vi "PH_Beckhoff.scale analog Beckhoff Value.vi"(0 "Beckhoff value":u32, 1 "Scaling Type":T1) -> (2 "DIM value":dbl)   [LabVIEW 2014, in "PH_Beckhoff.lvlib"]
doc: "This VI is forseen to scale the raw digital Beckhoff value to the DIM value to be published."
uses:
  PH_Beckhoff.lvlib
  PH_Beckhoff.Scaling Type.ctl
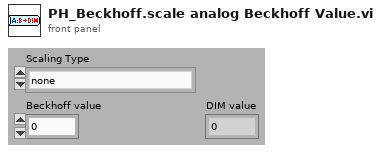
[diagram p1: front panel]
types:
  T1 = typedef "PH_Beckhoff.lvlib/PH_Beckhoff.Scaling Type.ctl" = enum16{"none", "0 ... 15 Bit -> 0 ... 5", "0 ... 15 Bit -> 0 ... 10", "0 ... 15 Bit -> 0 ... 25", "0 ... 15 Bit -> 4 ... 20", "0 ... 15 Bit -> 0 ... 1", "0 ... 15 Bit -> 0 ... 20000", "0 ... 15 Bit -> 0 ... 24000"}
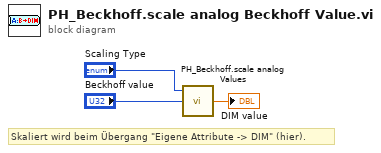
[diagram p0: block diagram]
diagram:
  # "Skaliert wird beim Übergang \"Eigene Attribute -> DIM\" (hier)."
  n1 = call "PH_Beckhoff.scale analog Values.vi"("Beckhoff value"="Beckhoff value", "Sca Type"="Scaling Type") -> ("Scaled DIM value"=→"DIM value":dbl)  [unwired: 1 in, 2 out]
